vi "Error Converter (ErrCode or Status).vi"(8 "error in (no error)":errorcluster caption="Fehler (Eingang, kein Fehler)", 11 "error code":i32 caption="Fehlercode") -> (0 "error out":errorcluster caption="Fehler (Ausgang)")   [LabVIEW 2021, in "labbCAN_Bus_API.lvlib"]
uses:
  labbCAN_Bus_API.lvlib
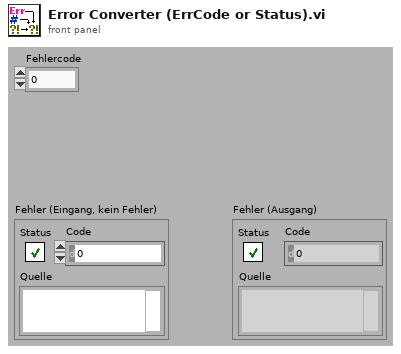
[diagram p1: front panel]
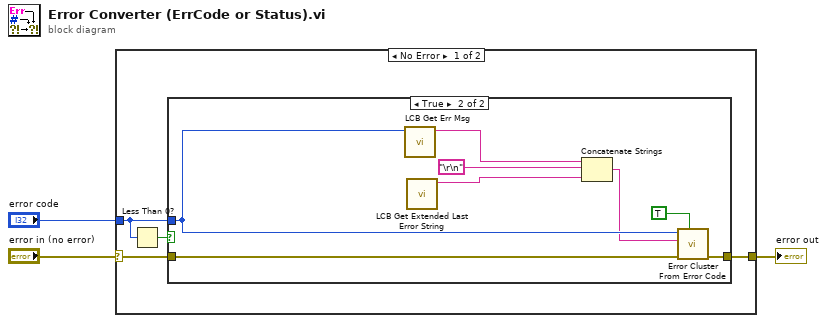
[diagram p0: block diagram]
diagram:
  n1 = case shown="No Error" "error in (no error)" {
    selector: "error in (no error)" -> [w6 w17]
    tunnel: [w4 w17] -> w2
    tunnel: "error code" -> [w5 _]
    frame No Error {
      n2 = Less Than 0?(x=w5) -> (x < 0?=w7:bool)
      n3 = case shown="True" w7 {
        tunnel: w6 -> [w8 w16]
        tunnel: w5 -> [_ w13]
        tunnel: [w8 w15] -> w4
        frame False {
        }
        frame True {
          n4 = call "LCB Get Err Msg.vi"("Error Code"=w13) -> ("Error Message"=w12:string)  [unwired: 9 in, 1 out]
          n5 = call "LCB Get Extended Last Error String.vi"() -> ("Error Message"=w10:string)  [unwired: 10 in, 1 out]
          n6 = Concatenate Strings(w12, "\r\n", w10) -> (w11:string)
          n7 = call <vilib>:"Error Cluster From Error Code.vi"("show call chain? (False)"=TRUE, "error in (no error)"=w16, "error message (\"\")"=w11, "error code (0)"=w13) -> ("error out"=w15:errorcluster)  [unwired: 5 in]
        }
      }
    }
    frame Error {
    }
  }
  "error out" <- w2
